vi "OpenFirstValidDevice.vi"(3 "error in (no error)":errorcluster, 5 "Device Keys":string[](array[string]), 6 "CmdLib In":refnum<k24>) -> (0 "error out":errorcluster, 1 "DeviceKey Out":string, 2 "CmdLib Out":refnum<k24>)   [LabVIEW 2013]
uses:
  C:/Code/Apps/Utilities/AG-UC2-UC8/AG-UC2-UC8/Install/Samples/LabVIEW/LabVIEW 2013/CmdLibAgilis.dll
  CmdLibAgilis.dll
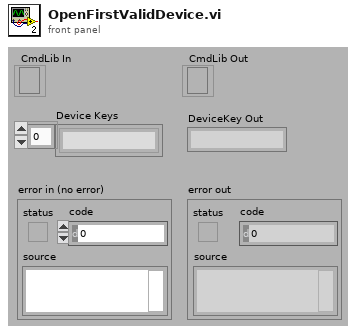
[diagram p1: front panel]
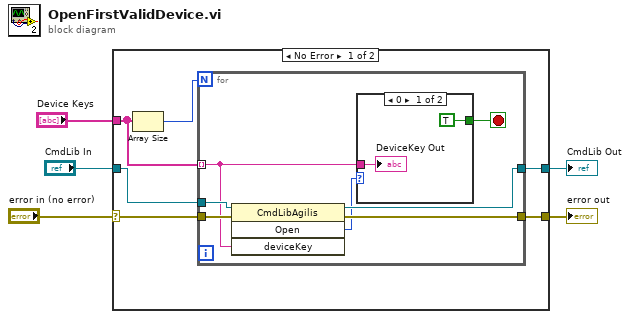
[diagram p0: block diagram]
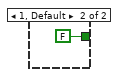
[diagram p2: hidden frame]
diagram:
  n1 = case shown="No Error" "error in (no error)" {
    selector: "error in (no error)" -> [w9 w23]
    tunnel: [w6 w23] -> w4
    tunnel: "CmdLib In" -> [w8 w22]
    tunnel: [w7 w22] -> w1
    tunnel: "Device Keys" -> [w10 _]
    frame No Error {
      n2 = Array Size(array=w10) -> (size(s)=w11:i32)
      n3 = for {
        N: w11 -> [_]
        tunnel: w10 -> [w13] mode=indexing
        tunnel: w9 -> [w18]
        tunnel: w8 -> [w17]
        tunnel: [w16] -> w7
        tunnel: [w15] -> w6
        stop <- w12 stop-if-true
        n4 = invoke class="CmdLibAgilis" method="Open"(reference=w17, error in=w18, "deviceKey"=w13) -> (reference out=w16:refnum<k24>, error out=w15:errorcluster, "Open"=w14:i32)  [unwired: 1 in, 1 out]
        n5 = case shown="0" w14 {
          tunnel: w13 -> [w20 _]
          tunnel: [TRUE FALSE] -> w12
          frame 0 {
            "DeviceKey Out" <- w20
          }
          frame 1, Default {
          }
        }
      }
    }
    frame Error {
    }
  }
  "error out" <- w4
  "CmdLib Out" <- w1
